vi "DeviceWriteArea.vi"(0 "Handle In":u64[](array[numeric]), 1 "AreaID":T1(ring), 2 "Address":u16=1, 3 "Amount":i32=1, 4 "BitArea":u8[](array[numeric]), 5 "WordArea":u16[](array[numeric]), 6 "error in (no error)":errorcluster) -> (12 "error out":errorcluster, 14 "Handle Out":u64[](array[numeric]), 15 "Result":i32)   [LabVIEW 2020, in "SnapMB.lvlib"]
uses:
  SnapMB.lvlib
  windows/snapmb.dll
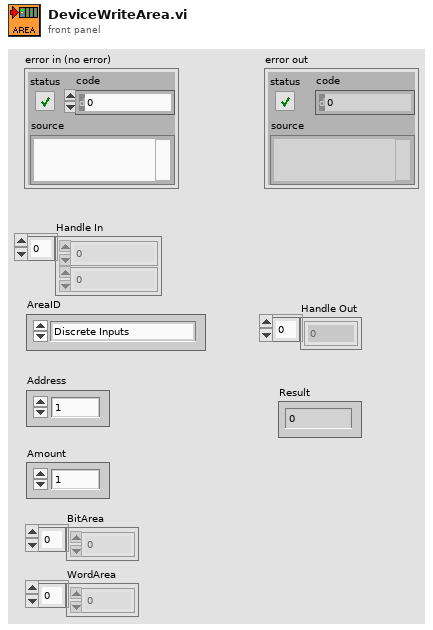
[diagram p1: front panel]
types:
  T1 = enum16{"Discrete Inputs", "Coils", "Input Registers", "Holding Registers"}
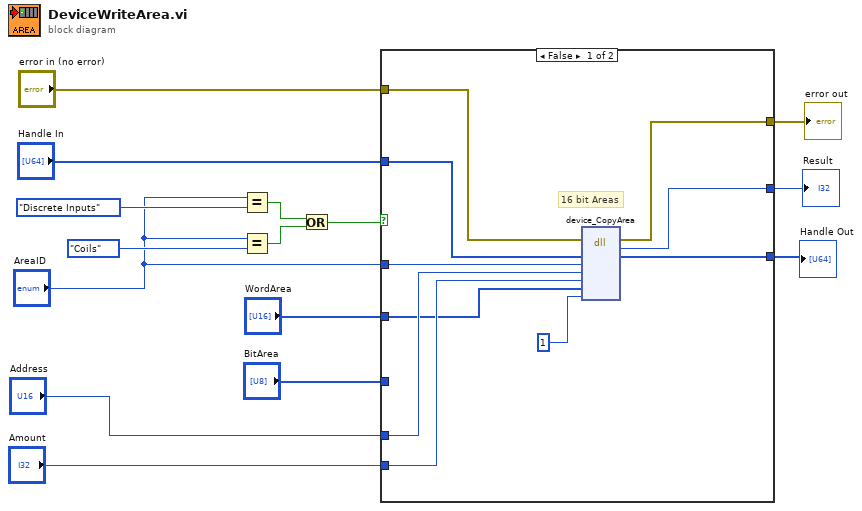
[diagram p0: block diagram]
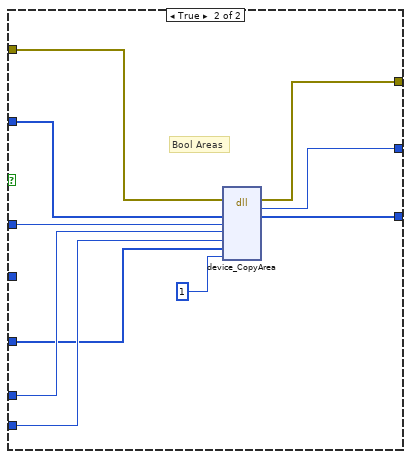
[diagram p2: hidden frame]
diagram:
  n1 = Equal?(x="AreaID", y=T1."Discrete Inputs") -> (x = y?=w13:bool)
  n2 = Equal?(x="AreaID", y=T1."Coils") -> (x = y?=w12:bool)
  n3 = Or(x=w13, y=w12) -> (x .or. y?=w11:bool)
  n4 = case shown="False" w11 {
    tunnel: "Handle In" -> [w25 w27]
    tunnel: "AreaID" -> [w24 w31]
    tunnel: "Amount" -> [w18 w29]
    tunnel: [w23 w32] -> w7
    tunnel: [w22 w33] -> w6
    tunnel: [w21 w34] -> w5
    tunnel: "error in (no error)" -> [w20 w35]
    tunnel: "Address" -> [w19 w30]
    tunnel: "WordArea" -> [w16 _]
    tunnel: "BitArea" -> [_ w26]
    frame False {
      # "16 bit Areas"
      n5 = dll-call lib="D:/SnapMB/LabView/lib/windows/snapmb.dll" fn="device_CopyArea"(error in=w20, "Device"=w25, "AreaID"=w24, "Address"=w19, "Amount"=w18, "Data"=w16, "CopyMode"=1) -> (error out=w21:errorcluster, "Result"=w22:i32, "Device"=w23:u64[])  [unwired: 7 in, 1 out]
    }
    frame True {
      # "Bool Areas"
      n6 = dll-call lib="D:/SnapMB/LabView/lib/windows/snapmb.dll" fn="device_CopyArea"(error in=w35, "Device"=w27, "AreaID"=w31, "Address"=w30, "Amount"=w29, "Data"=w26, "CopyMode"=1) -> (error out=w34:errorcluster, "Result"=w33:i32, "Device"=w32:u64[])  [unwired: 7 in, 1 out]
    }
  }
  "Handle Out" <- w7
  "Result" <- w6
  "error out" <- w5
